vi "Set X Y Positions.vi"(6 "Table Rotation":dbl, 8 "error in (no error)":errorcluster, 9 "Y Position":dbl, 10 "X Position":dbl, 11 "XRay Table in":refnum<class "XRay Table.lvclass">) -> (0 "error out":errorcluster, 3 "XRay Table out":refnum<class "XRay Table.lvclass">)   [LabVIEW 2026, in "XRay Table.lvclass"]
uses:
  XRay Table.lvclass
  XRay Table.lvclass/XRay Table.ctl
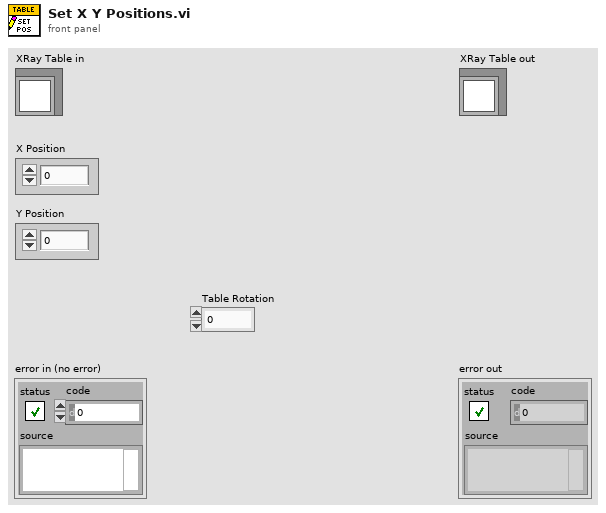
[diagram p1: front panel]
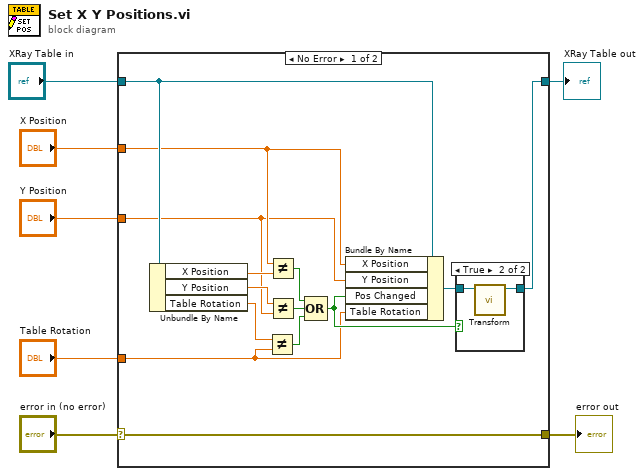
[diagram p0: block diagram]
diagram:
  n1 = case shown="No Error" "error in (no error)" {
    selector: "error in (no error)" -> [w21 w25]
    tunnel: [w21 w25] -> w6
    tunnel: [w19 w26] -> w4
    tunnel: "XRay Table in" -> [w18 w26]
    tunnel: "X Position" -> [w16 _]
    tunnel: "Y Position" -> [w14 _]
    tunnel: "Table Rotation" -> [w9 _]
    frame No Error {
      n2 = Unbundle By Name(w18) -> ("X Position"=w17:dbl, "Y Position"=w15:dbl, "Table Rotation"=w10:dbl)
      n3 = Not Equal?(x=w10, y=w9) -> (x != y?=w8:bool)
      n4 = Not Equal?(x=w16, y=w17) -> (x != y?=w13:bool)
      n5 = Not Equal?(x=w15, y=w14) -> (x != y?=w12:bool)
      n6 = Compound Arithmetic op=OR(w13, w12, w8) -> (w11:bool)
      n7 = Bundle By Name(cluster=w18, "X Position"=w16, "Y Position"=w14, "Pos Changed"=w11, "Table Rotation"=w9) -> (w20:refnum<class "XRay Table.lvclass">)
      n8 = case shown="True" w11 {
        tunnel: w20 -> [w22 w24]
        tunnel: [w22 w23] -> w19
        frame False {
        }
        frame True {
          n9 = call-dynamic "Transform.vi"("XRay Table in"=w24) -> ("XRay Table out"=w23:refnum<class "XRay Table.lvclass">)  [unwired: 9 in, 1 out]
        }
      }
    }
    frame Error {
    }
  }
  "error out" <- w6
  "XRay Table out" <- w4
